vi "MoreTestDataGFV.vi"() -> ()   [LabVIEW 2017]
uses:
  DatabaseContollerGFVenum.ctl
panel:
  out "data":i32
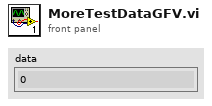
[diagram p1: front panel]
types:
  T1 = typedef "DatabaseContollerGFVenum.ctl" = enum16{"Get Objective Microns/Pixels", "Init and Open Database!", "Get User Name!", "Get Active Users Names!", "Get User Picture!", "Get User Phone Number!", "Get Setup Names!", "Get Active Microscope Objectives!", "Get Experiment Number!", "Get Sample Types!"}
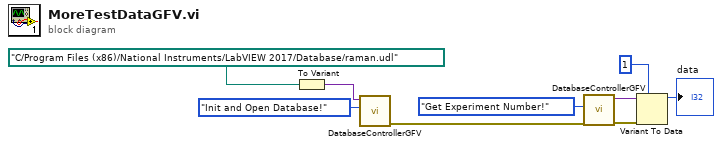
[diagram p0: block diagram]
diagram:
  n1 = To Variant(anything=path "C:/Program Files (x86)/National Instruments/LabVIEW 2017/Database/raman.udl" ("connection information")) -> (Variant=w2:variant)
  n2 = call "DatabaseControllerGFV.vi"("Enum"=DatabaseContollerGFVenum."Init and Open Database!", "Data in"=w2) -> ("error out"=w4:errorcluster)  [unwired: 8 in, 1 out]
  n3 = call "DatabaseControllerGFV.vi"("error in (no error)"=w4, "Enum"=DatabaseContollerGFVenum."Get Experiment Number!") -> ("error out"=w8:errorcluster, "Data Out"=w7:variant)  [unwired: 8 in]
  n4 = Variant To Data(error in=w8, type=1, Variant=w7) -> (data=→"data":i32)  [unwired: 1 out]
